vi "SetActualTemperature.vi"(8 "error in":T1, 11 "temperature in":sgl format="%#_g K") -> (0 "error out":T1, 3 "temperature":sgl format="%#_g K")   [LabVIEW 2016]
doc: "Sets a temperature between 0 and 300 Kelvin specified by the input \"temperature_in\". The input unit is Kelvin."
uses:
  Controls/Error_Out.ctl
  Files_ASC500/DLL/ASC500_RemoteControlV27.dll
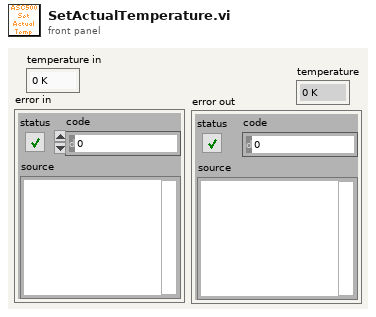
[diagram p1: front panel]
types:
  T1 = typedef "Error_Out.ctl" = errorcluster
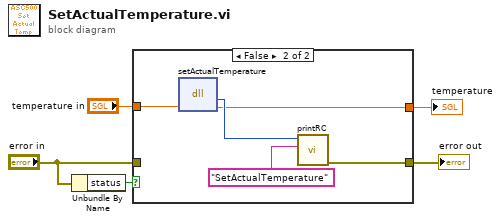
[diagram p0: block diagram]
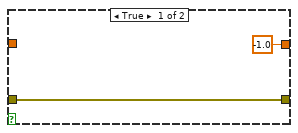
[diagram p2: hidden frame]
diagram:
  n1 = Unbundle By Name("error in") -> ("status"=w5:bool)
  n2 = case shown="False" w5 {
    tunnel: "error in" -> [w7 _]
    tunnel: [w7 w11] -> w3
    tunnel: "temperature in" -> [_ w10]
    tunnel: [sgl -1.0 ("temperature") w8] -> w1
    frame True {
    }
    frame False {
      n3 = dll-call lib="G:/SCMOperations/Share/ELE/Produkt Information/ASC500/04 Remote Control/02 development versions/2018Nov06/Files_ASC500/DLL/ASC500_RemoteControlV27.dll" fn="setActualTemperature"("temperature"=w10) -> ("return type"=w9:i32, "temperature"=w8:sgl)  [unwired: 3 in, 2 out]
      n4 = call "printRC.vi"("additional information"="SetActualTemperature", "RC"=w9) -> ("error out"=w11:T1)  [unwired: 9 in]
    }
  }
  "error out" <- w3
  "temperature" <- w1
